vi "novoGoleiroAlinharComABola.vi"(8 "balls":T1[](array[typedef]), 9 "Robot in":T2, 10 "Goleiro.X_padrao":dbl, 11 "IA State":T7={"our_robots"=[], "enemy_robots"=[], "balls"=[], "geometry"={"field_length"=0, "field_width"=0, "goal_width"=0, "goal_depth"=0, "center_circle_radius"=0, "defense_width"=0, "defense_depth"=0, "free_kick_from_defense_dist"=0, "penalty_spot_from_field_line_dist"=0, "penalty_line_from_spot_dist"=0, "half_moon_depth"=0, "half_moon_width"=0}, "IA Judge"={"stage"="", "command"="", "our_goalie_id"=0.0, "enemy_goalie_id"=0.0, "command enum"=enum."Halt", "Time"=enum."Azul"}, "Received Timestamp"=timestamp(0 s since 1904-01-01), "Events"={"Touch"=FALSE, "id touch"=0.0, "Ball out of \nVision"=FALSE, "Ball inside \nGoalie area"=FALSE, "Robot not responding"=FALSE, "Robots responding status"=[1.0, 1.0, 1.0, 1.0, 1.0, 1.0], "Enemy Ball \nPossession"=FALSE, "Id ini Possession"=0.0, "Ball Possesion"=FALSE, "Id Possesion"=0.0, "Ball at\nour goal side"=FALSE, "Ball at\ntouchline"=FALSE, "Ball at\nenemy goal side"=FALSE}}) -> (3 "Cluster de saída":T2)   [LabVIEW 2018]
uses:
  2019/VSS/Core/AI Input.ctl
  2019/VSS/Core/AI Robot.ctl
  2019/VSS/Intel/Functions Enum.ctl
  2019/VSS/Intel/AttackerStates.ctl
  2019/VSS/Path Planning/RRT/PathDests.ctl
  2019/VSS/Path Planning/RRT/PathDest.ctl
  2019/VSS/Core/AI Ball.ctl
  2019/VSS/Core/Field Size.ctl
  2019/VSS/Core/AI Judge.ctl
  2019/VSS/Intel/Command Enum.ctl
  2019/VSS/Util/Events/Events.ctl
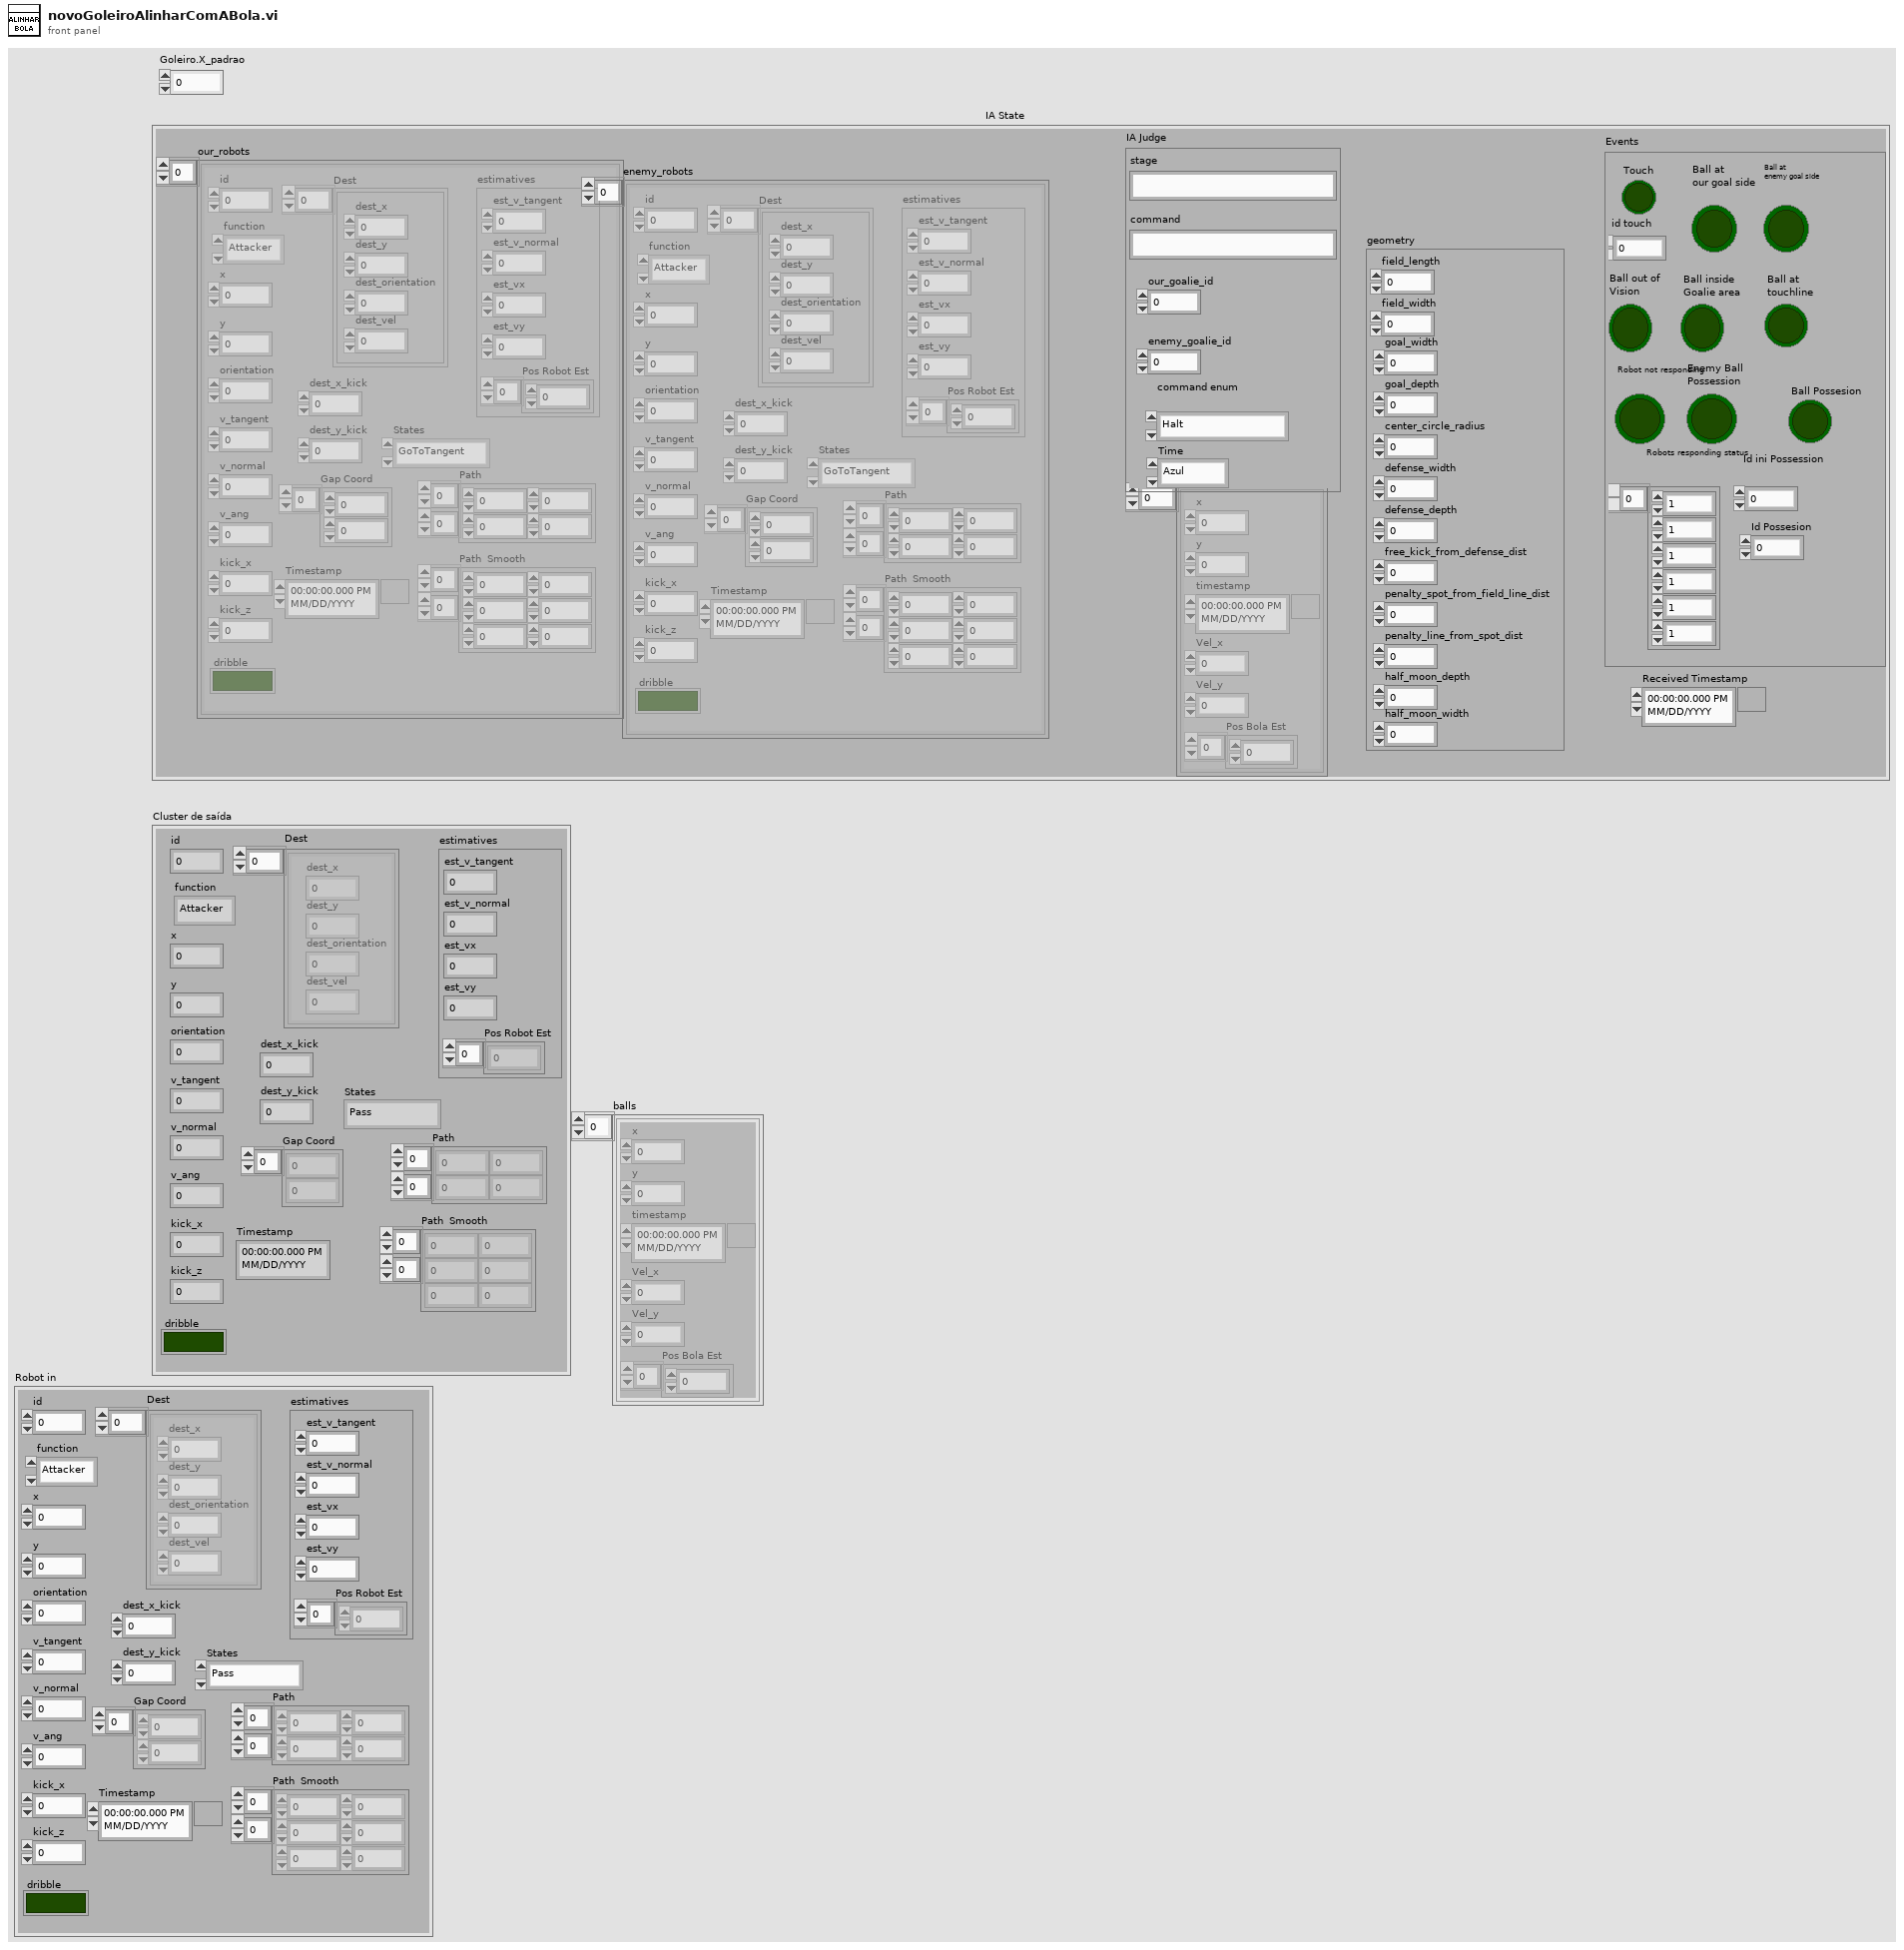
[diagram p1: front panel]
types:
  T1 = typedef "AI Ball.ctl" = cluster{"x":dbl, "y":dbl, "timestamp":timestamp, "Vel_x":dbl, "Vel_y":dbl, "Pos Bola Est":dbl[]}
  T2 = typedef "AI Robot.ctl" = cluster{"id":u32, "function":T3, "x":dbl, "y":dbl, "orientation":dbl, "v_tangent":dbl, "v_normal":dbl, "v_ang":dbl, "kick_x":dbl, "kick_z":dbl, "dribble":bool, "Timestamp":timestamp, "estimatives":cluster{"est_v_tangent":dbl, "est_v_normal":dbl, "est_vx":dbl, "est_vy":dbl, "Pos Robot Est":dbl[]}, "dest_x_kick":dbl, "dest_y_kick":dbl, "Gap Coord":dbl[], "States":T4, "Path ":dbl[][], "Path  Smooth":dbl[][], "Dest":T5}
  T3 = typedef "Functions Enum.ctl" = enum16{"Attacker", "Goalie", "Defender", "Striker", "Goto 0", "Dummy", "Kicker", "ZigZag"}
  T4 = typedef "AttackerStates.ctl" = enum16{"Pass", "GoToTangent", "BallGetting", "GoToKick", "Rotate anti-clockwise", "Rotate Clockwise", ""}
  T5 = typedef "PathDests.ctl" = T6[]
  T6 = typedef "PathDest.ctl" = cluster{"dest_x":dbl, "dest_y":dbl, "dest_orientation":dbl, "dest_vel":dbl}
  T7 = typedef "AI Input.ctl" = cluster{"our_robots":T2[], "enemy_robots":T2[], "balls":T1[], "geometry":T8, "IA Judge":T9, "Received Timestamp":timestamp, "Events":T11}
  T8 = typedef "Field Size.ctl" = cluster{"field_length":u32, "field_width":u32, "goal_width":u32, "goal_depth":u32, "center_circle_radius":u32, "defense_width":u32, "defense_depth":u32, "free_kick_from_defense_dist":u32, "penalty_spot_from_field_line_dist":u32, "penalty_line_from_spot_dist":u32, "half_moon_depth":u32, "half_moon_width":u32}
  T9 = typedef "AI Judge.ctl" = cluster{"stage":string, "command":string, "our_goalie_id":dbl, "enemy_goalie_id":dbl, "command enum":T10, "Time":enum16{"Azul", "Amarelo"}}
  T10 = typedef "Command Enum.ctl" = enum16{"Halt", "Stop", "Force Start", "PKA Normal Start", "Prepare Kickoff Ally", "PKE Normal Start", "Prepare Kickoff Enemy", "Prepare Penalty Ally", "PPA Normal Start", "Prepare Penalty Enemy", "PPE Normal Start", "Ball Placement Enemy Up", "Ball Placement Enemy Down", "Ball Placement Ally Up", "Ball Placement Ally Mid", "Ball Placement Ally Down", "Indirect Free Enemy", "Indirect Free Ally", "Timeout Enemy", "Timeout Ally", "Goal Enemy", "Goal Ally", "Normal Half Time", "Extra Time Break", "Extra Half Time", "None", "Post Game"}
  T11 = typedef "Events.ctl" = cluster{"Touch":bool, "id touch":dbl, "Ball out of \nVision":bool, "Ball inside \nGoalie area":bool, "Robot not responding":bool, "Robots responding status":dbl[], "Enemy Ball \nPossession":bool, "Id ini Possession":dbl, "Ball Possesion":bool, "Id Possesion":dbl, "Ball at\nour goal side":bool, "Ball at\ntouchline":bool, "Ball at\nenemy goal side":bool}
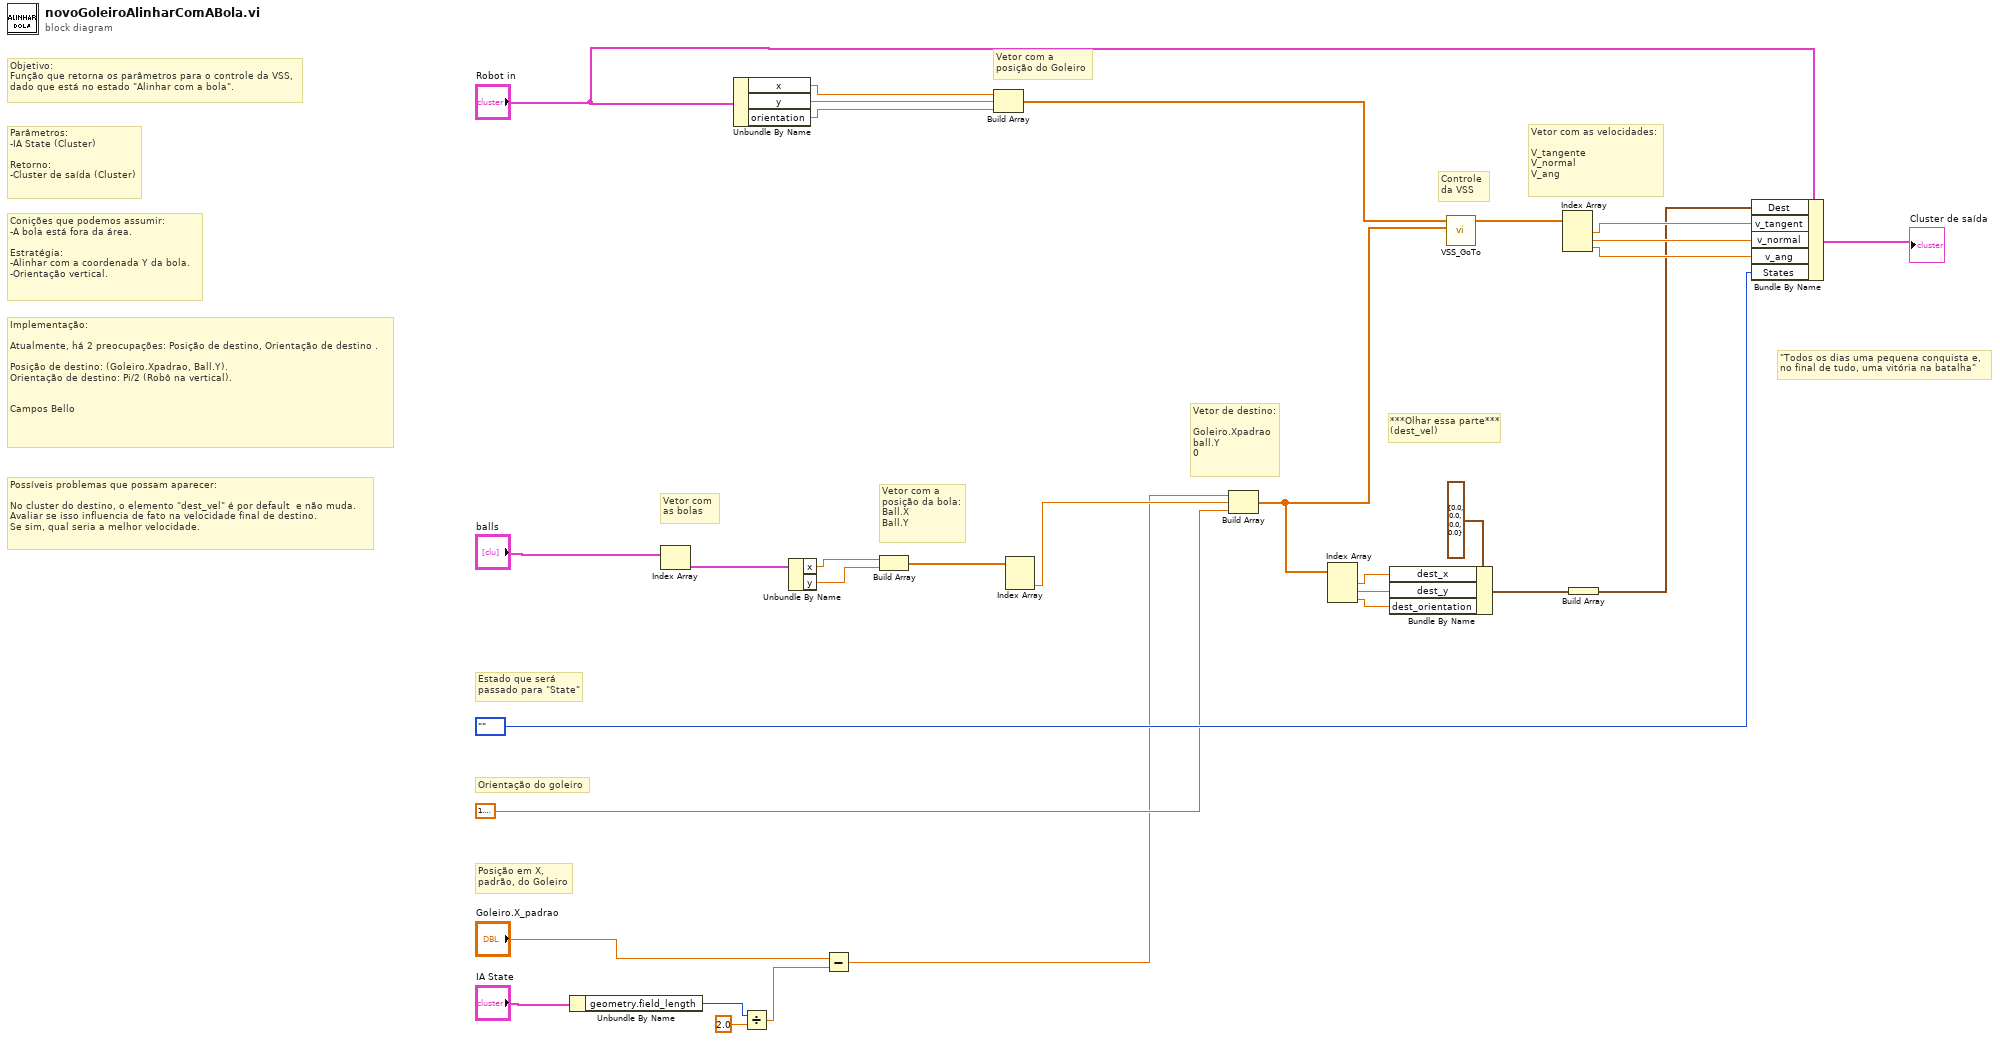
[diagram p0: block diagram]
diagram:
  # "\"Todos os dias uma pequena conquista e,\nno final de tudo, uma vitória na batalha\""
  # "Conições que podemos assumir:\n-A bola está fora da área.\n\nEstratégia:\n-Alinhar com a coordenada Y da bola.\n-Orientação vertical."
  # "Possíveis problemas que possam aparecer:\n\nNo cluster do destino, o elemento \"dest_vel\" é por default  e não muda. \nAvaliar se isso influencia de fato na velocidade final de destino.\nSe sim, qual seria a melhor velocidade."
  # "Implementação:\n\nAtualmente, há 2 preocupações: Posição de destino, Orientação de destino .\n\nPosição de destino: (Goleiro.Xpadrao, Ball.Y).\nOrientação de destino: Pi/2 (Robô na vertical).\n\n\nCampos Bello"
  # "Parâmetros:\n-IA State (Cluster)\n\nRetorno:\n-Cluster de saída (Cluster)"
  # "Objetivo:\nFunção que retorna os parâmetros para o controle da VSS,\ndado que está no estado \"Alinhar com a bola\"."
  # "Posição em X, \npadrão, do Goleiro"
  # "Orientação do goleiro"
  # "Estado que será\npassado para \"State\""
  # "Controle \nda VSS"
  # "***Olhar essa parte***\n(dest_vel)"
  # "Vetor com as velocidades:\n\nV_tangente\nV_normal\nV_ang"
  # "Vetor de destino:\n\nGoleiro.Xpadrao\nball.Y\n0"
  # "Vetor com a \nposição da bola:\nBall.X\nBall.Y"
  # "Vetor com \nas bolas"
  # "Vetor com a \nposição do Goleiro"
  n1 = Unbundle By Name("IA State") -> ("geometry.field_length"=w4:u32)
  n2 = Index Array(array="balls") -> (element=w31:T1)  [unwired: 1 in]
  n3 = Unbundle By Name("Robot in") -> ("x"=w10:dbl, "y"=w9:dbl, "orientation"=w8:dbl)
  n4 = Divide(x=w4, y=2.0) -> (x/y=w3:dbl)
  n5 = Unbundle By Name(w31) -> ("x"=w30:dbl, "y"=w29:dbl)
  n6 = Subtract(x="Goleiro.X_padrao", y=w3) -> (x-y=w1:dbl)
  n7 = Build Array(w30, w29) -> (w28:dbl[])
  n8 = Build Array(w10, w9, w8) -> (w27:dbl[])
  n9 = Index Array(array=w28) -> (element #2=w12:dbl)  [unwired: 2 in, 1 out]
  n10 = Build Array(w1, w12, 1.5707963267948966) -> (w21:dbl[])
  n11 = Index Array(array=w21) -> (element #1=w20:dbl, element #2=w19:dbl, element #3=w18:dbl)  [unwired: 3 in]
  n12 = Bundle By Name(cluster=T6 {"dest_x"=0.0, "dest_y"=0.0, "dest_orientation"=0.0, "dest_vel"=0.0} ("element"), "dest_x"=w20, "dest_y"=w19, "dest_orientation"=w18) -> (w17:T6)
  n13 = call "VSS_GoTo.vi"("SetPoint"=w21, "Position"=w27) -> ("Output Vel"=w26:dbl[])  [unwired: 9 in]
  n14 = Index Array(array=w26) -> (element #1=w25:dbl, element #2=w24:dbl, element #3=w23:dbl)  [unwired: 3 in]
  n15 = Build Array(w17) -> (w16:T6[])
  n16 = Bundle By Name(cluster="Robot in", "Dest"=w16, "v_tangent"=w25, "v_normal"=w24, "v_ang"=w23, "States"=AttackerStates."") -> (→"Cluster de saída":T2)
